vi "Read Analogue.vi"(8 "error in (no error)":errorcluster, 11 "Hioki BT4560B":refnum<class "Hioki BT4560B.lvclass">) -> (0 "error out":errorcluster, 2 "Measurement":dbl format="%.5f", 3 "Hioki BT4560B":refnum<class "Hioki BT4560B.lvclass">)   [LabVIEW 2019, in "Concrete.lvlib" / "Hioki BT4560B.lvclass"]
uses:
  Hioki BT4560B.lvclass
  Hioki BT4560B.lvclass/Hioki BT4560B.ctl
  Harware Abstraction/Analog In/Analog In.lvclass
  <instrlib>/HIOKI BT4560/HIOKI BT4560.lvlib
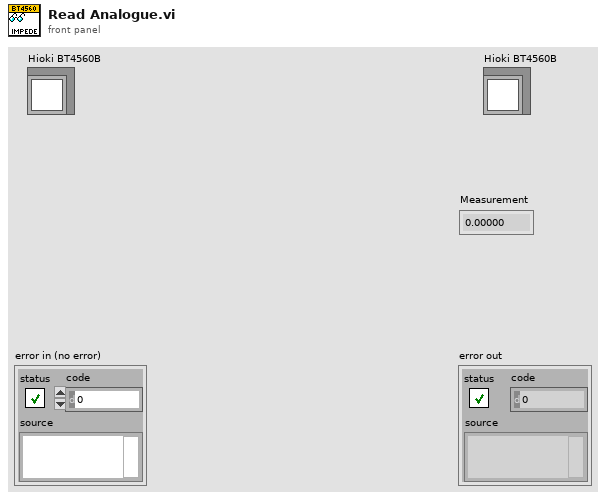
[diagram p1: front panel]
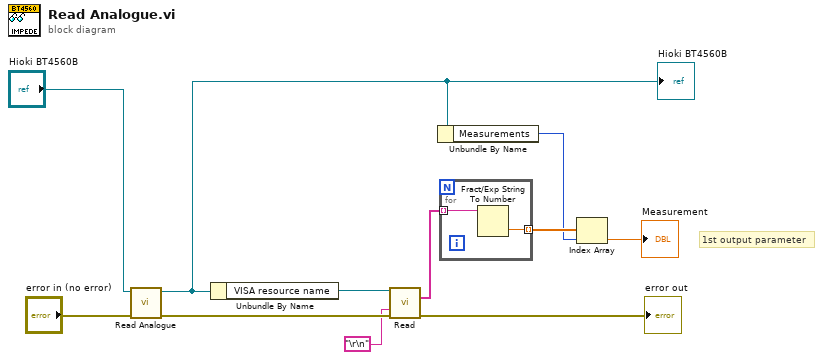
[diagram p0: block diagram]
diagram:
  # "1st output parameter"
  n1 = call-parent "Read Analogue.vi"("error in (no error)"="error in (no error)", "PS in"="Hioki BT4560B") -> ("error out"=w7:errorcluster, "PS out"=w1:refnum<class "Hioki BT4560B.lvclass">)  [unwired: 7 in, 1 out]
  "Hioki BT4560B" <- w1
  n2 = Unbundle By Name(w1) -> ("VISA resource name"=w5:refnum<visa-resource-name>)
  n3 = call <instrlib>:"Read.vi"("VISA session"=w5, "Terminator"="\r\n", "error in (no error)"=w7) -> ("Output Str"=w3:string[], "error out"=→"error out":errorcluster)  [unwired: 9 in, 2 out]
  n4 = Unbundle By Name(w1) -> ("Measurements"=w8:enum16{"Impedence", "Phase Angle", "OCV"})
  n5 = for {
    tunnel: w3 -> [w13] mode=indexing
    tunnel: [w12] -> w9 mode=indexing
    n6 = Fract/Exp String To Number(string=w13) -> (number=w12:dbl)  [unwired: 3 in, 1 out]
  }
  n7 = Index Array(array=w9, index=w8) -> (element=→"Measurement":dbl)
